vi "Read_Chan_Value_Gen.vi"(10 "Desired Ch Names":string[](array[string]), 11 "Raw data file":path) -> (2 "Values":string[](array[string]))   [LabVIEW 2011]
uses:
  Globals/Meas_global.vi
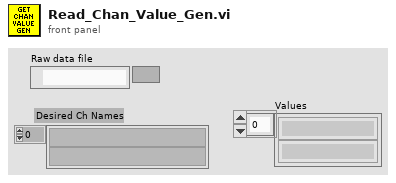
[diagram p1: front panel]
types:
  T1 = typedef "Post_Process.ctl" = enum16{"Take New Data", "Post Process Raw Data File"}
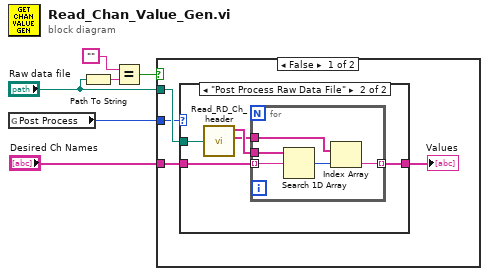
[diagram p0: block diagram]
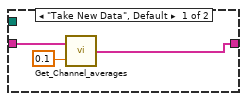
[diagram p2: hidden frame]
diagram:
  n1 = global read "Meas_global.vi" "Post Process"() -> (w6:T1)
  n2 = Path To String(path="Raw data file") -> (string=w2:string)
  n3 = Equal?(x="", y=w2) -> (x = y?=w4:bool)
  n4 = case shown="False" w4 {
    tunnel: "Raw data file" -> [w10 _]
    tunnel: w6 -> [w9 _]
    tunnel: "Desired Ch Names" -> [w7 _]
    frame False {
      n5 = case shown="\"Post Process Raw Data File\"" w9 {
        tunnel: w10 -> [_ w18]
        tunnel: [w12 w14] -> w8
        tunnel: w7 -> [w11 w15]
        frame "Take New Data", Default {
          n6 = call "Get_Channel_averages.vi"("Desired Ch Names"=w11, "Averaging time (mins)"=0.1) -> ("Values"=w12:string[])  [unwired: 1 in, 2 out]
        }
        frame "Post Process Raw Data File" {
          n7 = call "Read_RD_Ch_header.vi"("Raw data file"=w18) -> ("Ch Name Out"=w17:string[], "Ch Values"=w16:string[])  [unwired: 2 out]
          n8 = for {
            tunnel: w17 -> [w23]
            tunnel: w16 -> [w22]
            tunnel: w15 -> [w20] mode=indexing
            tunnel: [w19] -> w14 mode=indexing
            n9 = Search 1D Array(1D array=w23, element=w20) -> (index of element=w21:i32)  [unwired: 1 in]
            n10 = Index Array(array=w22, index=w21) -> (element=w19:string)
          }
        }
      }
      "Values" <- w8
    }
    frame True {
    }
  }
